vi "Password_Authentication_(SubVI).vi"(11 "String":string) -> (2 "True / False":bool=TRUE, 3 "Access Status":string)   [LabVIEW 2017]
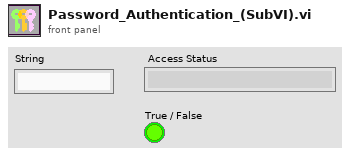
[diagram p1: front panel]
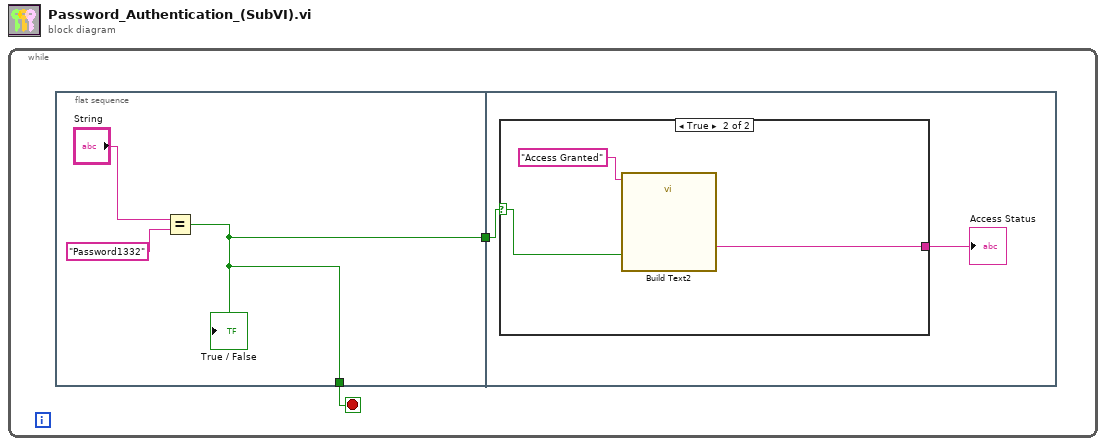
[diagram p0: block diagram]
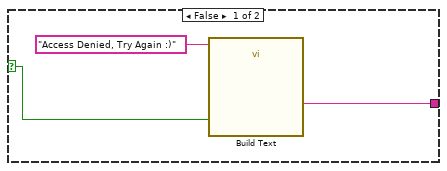
[diagram p2: hidden frame]
diagram:
  n1 = while {
    stop <- w1 stop-if-true
    n2 = flat-sequence {
      tunnel: [w4] -> w2
      tunnel: [w4] -> w1
      tunnel: w2 -> [w7]
      frame #0 {
        n3 = Equal?(x="String", y="Password1332") -> (x = y?=w4:bool)
        "True / False" <- w4
      }
      frame #1 {
        n4 = case shown="True" w7 {
          selector: w7 -> [w8 w11]
          tunnel: [w10 w13] -> w6
          frame False {
            n5 = call "Build Text"("Beginning Text"="Access Denied, Try Again :)", "Access Denied, Try Again :)"=w8) -> ("Result"=w10:string)  [unwired: 12 in, 1 out]
          }
          frame True {
            n6 = call "Build Text2"("Beginning Text"="Access Granted", "Access Granted"=w11) -> ("Result"=w13:string)  [unwired: 12 in, 1 out]
          }
        }
        "Access Status" <- w6
      }
    }
  }
